vi "Set Magnet Field.vi"(4 "Mode":T2, 6 "Axis":T1, 8 "error in (no error)":errorcluster, 9 "Target Rate (T/min)":dbl, 10 "Target Field (T)":dbl, 11 "Instrument.Oxford1820 in":refnum<class "Instrument.Oxford1820.lvclass">) -> (0 "error out":errorcluster, 3 "Instrument.Oxford1820 out":refnum<class "Instrument.Oxford1820.lvclass">)   [LabVIEW 2016, in "Instrument.Oxford1820.lvclass"]
uses:
  Instrument.Oxford1820.lvclass
  <userlib>/LevyLab/Levylab Instruments/Instrument Types/Cryostat/Typedefs/Magnet Mode--Enum.ctl
  <userlib>/LevyLab/Levylab Instruments/Instrument Types/Cryostat/Typedefs/Magnet Axis--Enum.ctl
  Typedefs/Instrument.Oxford1820.Commands-enum.ctl
  Typedefs/Instrument.Oxford1820.setMagnet-cluster.ctl
  Typedefs/Targets.ctl
  <userlib>/LevyLab/Levylab Instruments/Instrument Types/Cryostat/Instrument.Cryostat.lvclass
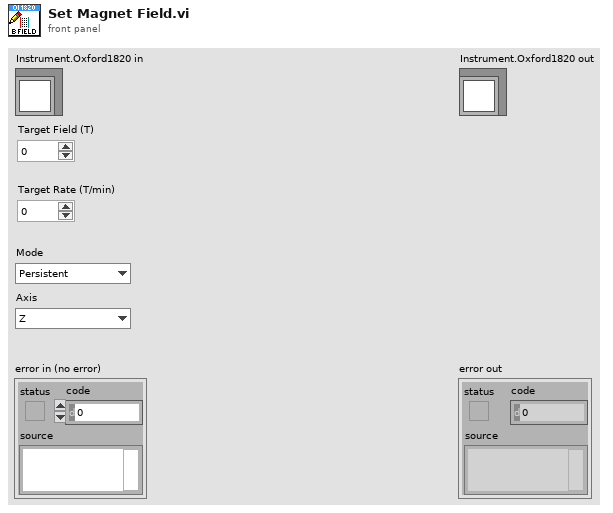
[diagram p1: front panel]
types:
  T1 = typedef "Instrument.Cryostat.lvclass/Magnet Axis--Enum.ctl" = enum16{"Z", "X", "Y"}
  T2 = typedef "Instrument.Cryostat.lvclass/Magnet Mode--Enum.ctl" = enum16{"Persistent", "Driven"}
  T3 = typedef "Instrument.Oxford1820.lvclass/Targets.ctl" = cluster{"Field (T)":dbl, "Field Rate (T/min)":dbl}
  T4 = typedef "Instrument.Oxford1820.lvclass/Instrument.Oxford1820.setMagnet-cluster.ctl" = cluster{"Target":T3, "persistent mode":bool}
  T5 = typedef "Instrument.Oxford1820.lvclass/Instrument.Oxford1820.Commands-enum.ctl" = enum16{"setAction", "setTarget", "setSwitchHeat", "setLambda", "setFillMode", "setNeedleValve", "setMagnetField", "getStatus", "getTarget", "getSwitchHeat", "getPSUField", "newcommand", "getMagnetField"}
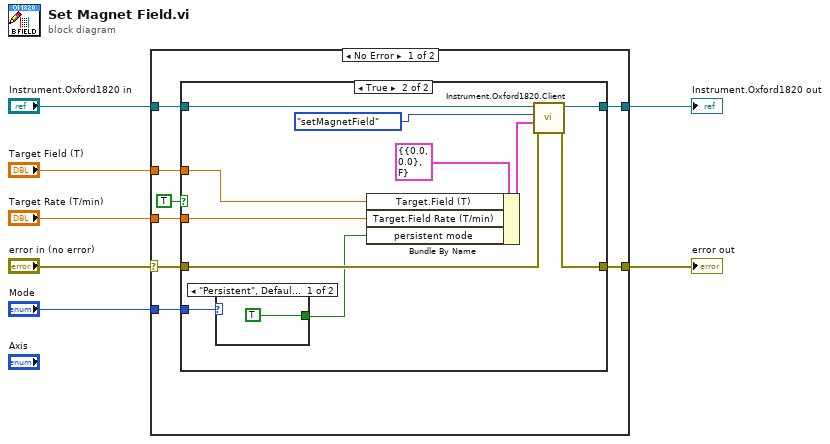
[diagram p0: block diagram]
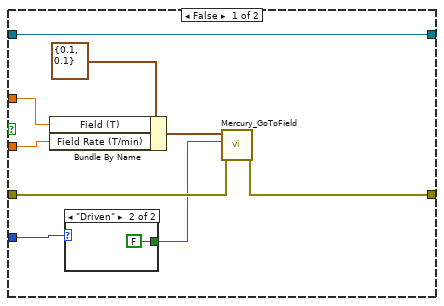
[diagram p2: hidden frame]
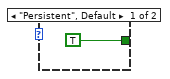
[diagram p3: hidden frame]
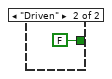
[diagram p4: hidden frame]
diagram:
  n1 = case shown="No Error" "error in (no error)" {
    selector: "error in (no error)" -> [w10 w41]
    tunnel: "Mode" -> [w15 _]
    tunnel: "Target Rate (T/min)" -> [w14 _]
    tunnel: [w9 w41] -> w5
    tunnel: "Target Field (T)" -> [w13 _]
    tunnel: "Instrument.Oxford1820 in" -> [w12 w40]
    tunnel: [w11 w40] -> w1
    frame No Error {
      n2 = case shown="True" TRUE {
        tunnel: w15 -> [w20 w37]
        tunnel: w14 -> [w17 w36]
        tunnel: w13 -> [w18 w35]
        tunnel: w12 -> [w16 w34]
        tunnel: [w16 w33] -> w11
        tunnel: w10 -> [w24 w32]
        tunnel: [w23 w30] -> w9
        frame False {
          n3 = Bundle By Name(cluster=T3 {"Field (T)"=0.1, "Field Rate (T/min)"=0.1} ("Mercury Targets"), "Field (T)"=w18, "Field Rate (T/min)"=w17) -> (w21:T3)
          n4 = case shown="\"Driven\"" w20 {
            tunnel: [TRUE ("persistent mode") FALSE ("persistent mode")] -> w19
            frame "Persistent", Default {
            }
            frame "Driven" {
            }
          }
          n5 = call "Mercury_GoToField.vi"("error in"=w24, "persistent mode"=w19, "Mercury Targets"=w21) -> ("error out"=w23:errorcluster)  [unwired: 8 in]
        }
        frame True {
          n6 = case shown="\"Persistent\", Default" w37 {
            tunnel: [TRUE ("persistent mode") FALSE ("persistent mode")] -> w28
            frame "Persistent", Default {
            }
            frame "Driven" {
            }
          }
          n7 = Bundle By Name(cluster=T4 {"Target"={"Field (T)"=0.0, "Field Rate (T/min)"=0.0}, "persistent mode"=FALSE} ("output cluster"), "Target.Field (T)"=w35, "Target.Field Rate (T/min)"=w36, "persistent mode"=w28) -> (w29:T4)
          n8 = call "Instrument.Oxford1820.Client.vi"("error in (no error)"=w32, "Data"=w29, "Commands"=Instrument.Oxford1820.Commands-enum."setMagnetField", "Instrument.1820 in"=w34) -> ("error out"=w30:errorcluster, "Instrument.1820 out"=w33:refnum<class "Instrument.Oxford1820.lvclass">)  [unwired: 5 in, 1 out]
        }
      }
    }
    frame Error {
    }
  }
  "Instrument.Oxford1820 out" <- w1
  "error out" <- w5
